vi "Teleop.vi"(10 "Match Info":T2={"Autonomous Elapsed Seconds"=0.0, "TeleOp Elapsed Seconds"=0.0, "Disabled Elapsed Seconds"=0.0, "Visited Autonomous"=FALSE, "Visited TeleOp"=FALSE, "Visited Disabled"=FALSE, "Autonomous Settings"={"Autonomous Style"=enum."Independent", "VI Refnum"=refnum}}, 11 "Call Context":T3) -> ()   [LabVIEW 2016]
doc: "This VI is called for each TeleOp packet received from the DS where the robot is not disabled. It is often used to read from the joysticks and update I/O or to update setpoints for timed control loops. It should complete and return within 20 milliseconds or it may miss DS packets."
uses:
  <vilib>/Rock Robotics/WPI/DriverStation/WPI_DriverStationDerivedRobotMode.ctl
  <vilib>/Rock Robotics/WPI/DriverStation/WPI_DriverStationMatch Info.ctl
  Typedefs/typedef_cluster_Teleop Local Data.ctl
  Typedefs/typedef_enum_Teleop State.ctl
  Typedefs/typedef_enum_Joystick Buttons.ctl
  Robot Global Data.vi
  <vilib>/Rock Robotics/WPI/Utilities/WPI_GetSetVariantRefNum.vi
  <vilib>/Rock Robotics/Network Tables/NT Read Boolean.vi
  <vilib>/Rock Robotics/Network Tables/NT Write Boolean.vi
  <vilib>/Rock Robotics/Network Tables/NT Read Number.vi
  <vilib>/Rock Robotics/WPI/Ultrasonic/WPI_SonarSRF04DigitalRefNum Registry Get.vi
  <vilib>/Rock Robotics/WPI/Ultrasonic/WPI_SonarSRF04DigitalGetRange.vi
panel:
  out "error out":errorcluster
  out "Teleop Local Data out":T1 {"Drive Twist" format="%.2f"; "Drive Forward" format="%.2f"; "Flywheel" format="%.2f"; "Outlet Flap" format="%_4p"; "Inlet Flap" format="%_4p"; "Camera Angle" format="%_4p"; "Collect Motor" format="%_4p"; "Climb Motor" format="%.3f"; "Accel_Y" format="%.3f"; "Accel_X" format="%.3f"; "Obj_deg_Up" format="%.4f"; "Obj_deg_Rt" format="%.1f"; "dT" format="%.4f"}
  out "Sample Slider 0":dbl(slide) scale=0.0..5.0
  out "Sample Boolean 1":bool
  out "Sample Boolean 0":bool
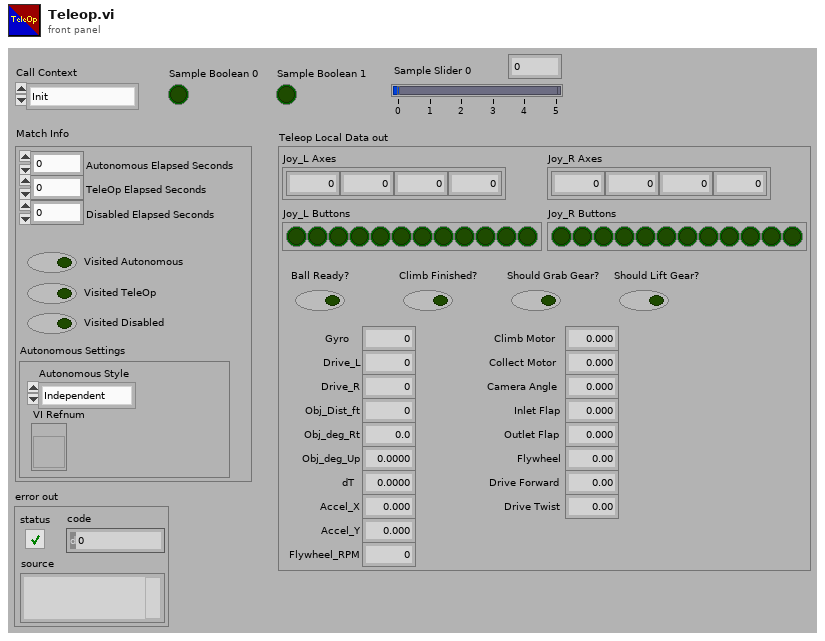
[diagram p1: front panel]
types:
  T1 = typedef "typedef_cluster_Teleop Local Data.ctl" = cluster{"Joy_L Axes":dbl[], "Joy_L Buttons":bool[], "Joy_R Axes":dbl[], "Joy_R Buttons":bool[], "Gyro":dbl, "Drive_L":i32, "Drive_R":i32, "Obj_Dist_ft":dbl, "Obj_deg_Rt":dbl, "Obj_deg_Up":dbl, "dT":dbl, "Accel_X":dbl, "Accel_Y":dbl, "Flywheel_RPM":dbl, "Ball Ready?":bool, "Climb Finished?":bool, "Should Grab Gear?":bool, "Should Lift Gear?":bool, "Climb Motor":dbl, "Collect Motor":dbl, "Camera Angle":dbl, "Inlet Flap":dbl, "Outlet Flap":dbl, "Flywheel":dbl, "Drive Forward":dbl, "Drive Twist":dbl}
  T2 = typedef "WPI_DriverStationMatch Info.ctl" = cluster{"Autonomous Elapsed Seconds":dbl, "TeleOp Elapsed Seconds":dbl, "Disabled Elapsed Seconds":dbl, "Visited Autonomous":bool, "Visited TeleOp":bool, "Visited Disabled":bool, "Autonomous Settings":cluster{"Autonomous Style":enum16{"Iterative", "Independent"}, "VI Refnum":refnum<vi>}}
  T3 = typedef "WPI_DriverStationDerivedRobotMode.ctl" = enum16{"Init", "Execute", "Stop"}
  T4 = typedef "typedef_enum_Teleop State.ctl" = enum16{"StartTeleop", "In Joy_L", "In Joy_R", "In Accel", "In Gyro", "In Drive_L", "In Drive_R", "In Fly_RPMs", "In Switch_Ball", "In Switch_Climbed", "In Get Vision Result", "Calc dT", "Calc Grabber", "Calc Lifter", "Calc Climb", "Calc Collect", "Calc Cam_Angle", "Calc Inlet_Flap", "Calc Outlet_Flap", "Calc Flywheel", "Calc Drive_Forward", "Calc Drive_Twist", "Out Drive_Forward", "Out Drive_Twist", "Out Flywheel", "Out Grabber", "Out Lifter", "Out Climb", "Out Collect", "Out Cam_Angle", "Out Inlet_Flap", "Out Outlet_Flap", "End Teleop"}
  T5 = typedef "typedef_enum_Joystick Buttons.ctl" = enum16{"Trigger", "Thumb", "Top3", "Top4", "Top5", "Top6", "Low7", "Low8", "Low9", "Low10", "Low11", "Low12", "Hat0", "Hat1", "Hat2", "Hat3", "Hat4", "Hat5", "Hat6", "Hat7", "Hat8"}
  T6 = typedef "WPI_JoystickDevRef.ctl" = cluster{"Device":T7}
  T7 = typedef "WPI_JoystickDeviceEnum.ctl" = enum16{"USB 0", "USB 1", "USB 2", "USB 3", "USB 4", "USB 5"}
  T8 = typedef "WPI_AccelerometerDevRef.ctl" = cluster{"DevStatus":errorcluster, "Scaling":T9, "Analog Channels":T10, "I2C Bus":T12, "SPI Bus":T13, "Accel Range":T14, "ADXL Axes":T15, "Handle":i32, "Device Address":u8, "Accel Type":enum16{"Analog", "ADXL345 I2C", "ADXL345 SPI", "Internal", "ADXL362 SPI"}}
  T9 = typedef "WPI_AccelerometerScaling.ctl" = cluster{"Gain (VoltsPerG)":dbl, "Center Voltage":dbl}
  T10 = typedef "WPI_AccelerometerAnalogChannels.ctl" = cluster{"X-Axis":T11, "Y-Axis":T11, "Z-Axis":T11}
  T11 = typedef "FPGA_AIChannel.ctl" = enum8{"AI 0", "AI 1", "AI 2", "AI 3", "AI MXP 0", "AI MXP 1", "AI MXP 2", "AI MXP 3", "Invalid"}
  T12 = typedef "i2c_bus.ctl" = enum16{"I2C On-Board", "I2C MXP", "Invalid"}
  T13 = typedef "spi_bus.ctl" = enum16{"SPI On-Board, CS0", "SPI On-Board, CS1", "SPI On-Board, CS2", "SPI On-Board, CS3", "SPI MXP", "Invalid"}
  T14 = typedef "ADXL345 Range.ctl" = u8
  T15 = typedef "WPI_AccelerometerADXL345 Axes.ctl" = cluster{"X-Axis":bool, "Y-Axis":bool, "Z-Axis":bool}
  T16 = cluster{"X-Axis":dbl, "Y-Axis":dbl, "Z-Axis":dbl}
  T17 = typedef "WPI_GyroDevRef.ctl" = cluster{"DevStatus":errorcluster, "Analog Channel":T11, "Offset":dbl, "Gain (VoltsPerDegree/Second)":dbl, "Gyro Type":enum16{"Analog", "XRS450"}, "Handle":i32, "SPI Bus":T13, "Device Found":bool, "Sample Rate":dbl, "Calibrate On Open":bool}
  T18 = typedef "WPI_MotorControlDeviceRef.ctl" = cluster{"DeviceStatus":errorcluster, "Type":T19, "PWM":cluster{"PWM Channel":T20, "DeadBand":T21}, "CAN":cluster{"Device Number":u8, "SetOutput VI Ref":variant, "GetOutput VI Ref":variant, "Enable VI Ref":variant, "Disable VI Ref":variant, "Data":variant}, "Invert":bool}
  T19 = typedef "WPI_MotorControlType.ctl" = enum16{"PWM", "CAN"}
  T20 = typedef "FPGA_DIOPWMChannel.ctl" = enum8{"PWM 0", "PWM 1", "PWM 2", "PWM 3", "PWM 4", "PWM 5", "PWM 6", "PWM 7", "PWM 8", "PWM 9", "PWM MXP 0", "PWM MXP 1", "PWM MXP 2", "PWM MXP 3", "PWM MXP 4", "PWM MXP 5", "PWM MXP 6", "PWM MXP 7", "PWM MXP 8", "PWM MXP 9", "Invalid"}
  T21 = typedef "WPI_PWMDeadband.ctl" = cluster{"Name":string, "maxPositivePwm":i32, "minPositivePwm":i32, "centerPwm":i32, "maxNegativePwm":i32, "minNegativePwm":i32, "angularRange":u16}
  T22 = typedef "WPI_CANTalonSRX_GlobalStatus.ctl" = cluster{"Applied Throttle":dbl, "Module Enabled":bool, "CAN Error":errorcluster, "Closed Loop Error":dbl, "Forward Limit Switch Closed":bool, "Reverse Limit Switch Closed":bool, "Sensor Position":dbl, "Sensor Velocity":dbl, "Current":dbl, "Sticky Fault - Over Temp":bool, "Sticky Fault - Under Voltage":bool, "Sticky Fault - Forward Limit":bool, "Sticky Fault - Reverse Limit":bool, "Sticky Fault - Forward Soft Limit":bool, "Sticky Fault - Reverse Soft Limit":bool, "Brake is Enabled":bool, "Encoder Position":dbl, "Encoder Velocity":dbl, "Encoder Index Count":dbl, "Encoder A Pin State":bool, "Encoder B Pin State":bool, "Encoder Index Pin State":bool, "Analog In":dbl, "Analog In Velocity":dbl, "Temperature (C)":dbl, "Battery Voltage":dbl, "Control 5 Is Supported":bool, "Current Profile Slot Select":dbl, "Pos Div 8":bool, "Vel Div 4":bool, "Pulse Width Position":i32, "Pulse Width Velocity":i32, "Pulse Width Rise To Rise (us)":i32, "Pulse Width Rise To Fall (us)":i32, "Mot Prof Active Is Under Run":bool, "Mot Prof Active Has Under Run":bool, "Mot Prof Active Is Last":bool, "Mot Prof Active Velocity Only":bool, "Mot Prof Active Is Valid":bool, "Mot Prof Buffer Is Full":bool, "Mot Prof Active Profile Slot Select":i32, "Mot Prof NextID":i32, "Mot Prof Count":i32, "Mot Prof Active Velocity":dbl, "Mot Prof Active Position":dbl, "Mot Prof Output Enable":i32}
  T23 = typedef "WPI_UltrasonicDeviceRef.ctl" = cluster{"DevStatus":errorcluster, "Ping Channel":T24, "Echo Channel":T24, "CntIndex":T25}
  T24 = typedef "FPGA_DIOChannel.ctl" = enum8{"DIO 0", "DIO 1", "DIO 2", "DIO 3", "DIO 4", "DIO 5", "DIO 6", "DIO 7", "DIO 8", "DIO 9", "DIO MXP 0", "DIO MXP 1", "DIO MXP 2", "DIO MXP 3", "DIO MXP 4", "DIO MXP 5", "DIO MXP 6", "DIO MXP 7", "DIO MXP 8", "DIO MXP 9", "DIO MXP 10", "DIO MXP 11", "DIO MXP 12", "DIO MXP 13", "DIO MXP 14", "DIO MXP 15", "SPI Port CS1", "SPI Port CS2", "SPI Port CS3", "SPI Port MISO", "SPI Port MOSI", "Invalid"}
  T25 = typedef "FPGA_CounterCtrSystemIndex.ctl" = enum8{"Ctr 0", "Ctr 1", "Ctr 2", "Ctr 3", "Ctr 4", "Ctr 5", "Ctr 6", "Ctr 7", "Invalid"}
  T26 = typedef "WPI_DigitalInputDevRef.ctl" = cluster{"DevStatus":errorcluster, "DIO Channel":T24}
  T27 = typedef "typedef_cluster_Object Params.ctl" = cluster{"Dist_ft":dbl, "Deg_Rt":dbl, "Deg_Up":dbl, "Cam_FPS":dbl}
  T28 = typedef "WPI_ServoDeviceRef.ctl" = cluster{"DeviceStatus":errorcluster, "PWM Channel":T20, "DeadBand":T21}
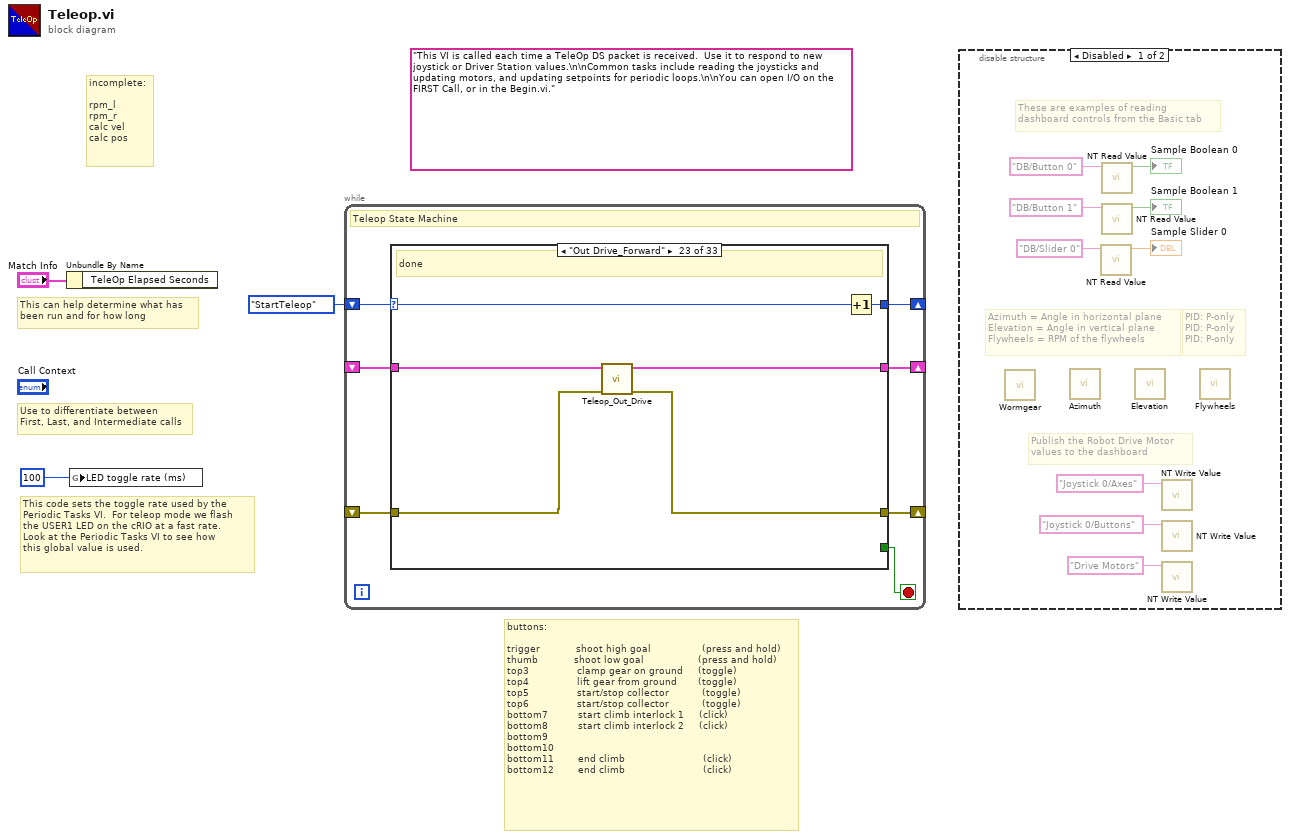
[diagram p0: block diagram]
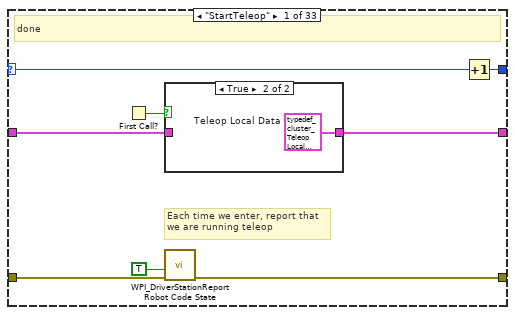
[diagram p3: hidden frame]
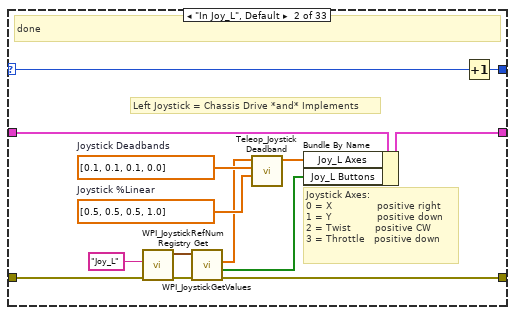
[diagram p5: hidden frame]
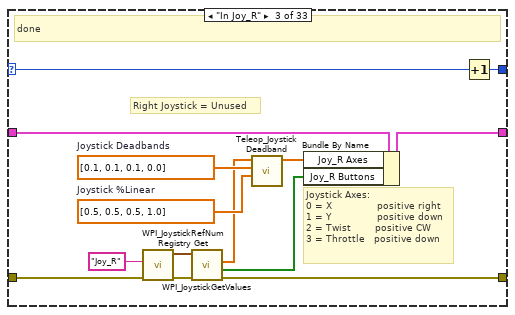
[diagram p6: hidden frame]
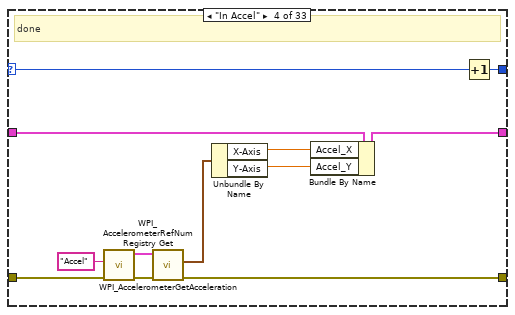
[diagram p7: hidden frame]
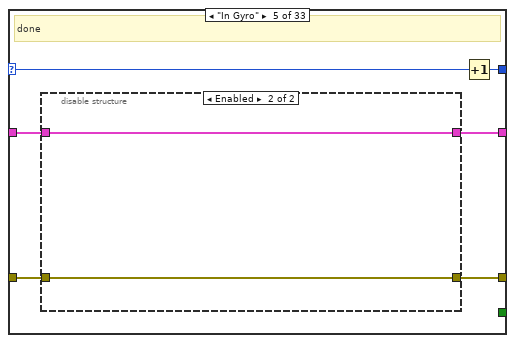
[diagram p8: hidden frame]
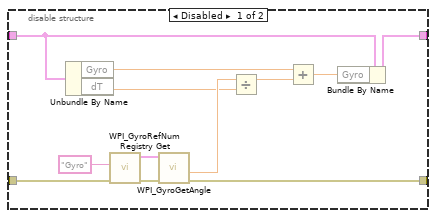
[diagram p9: hidden frame]
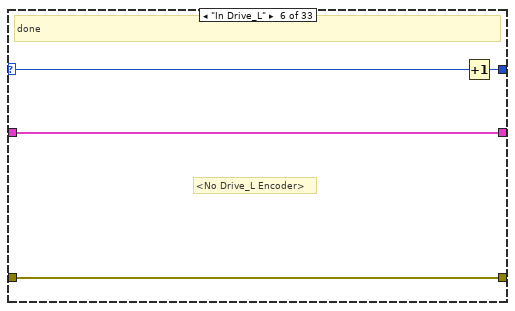
[diagram p10: hidden frame]
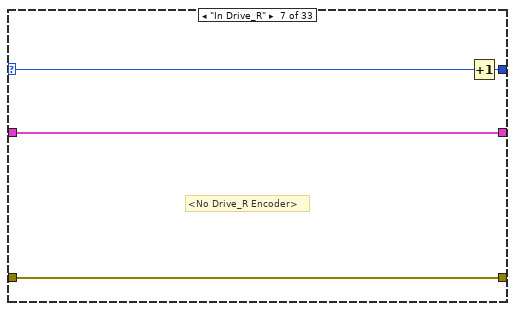
[diagram p11: hidden frame]
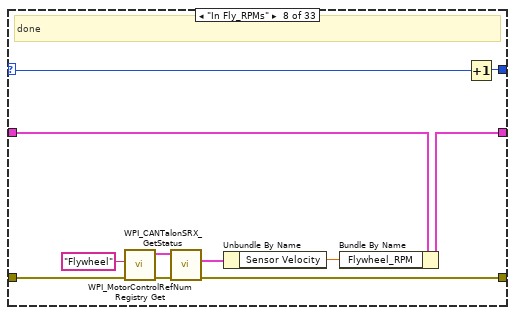
[diagram p12: hidden frame]
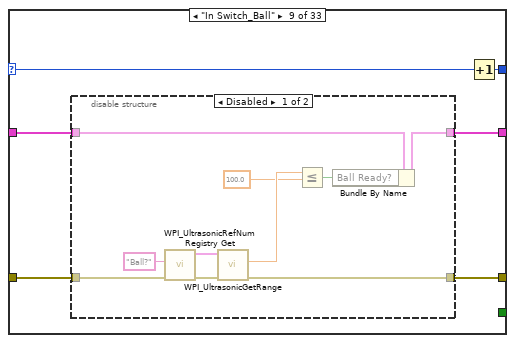
[diagram p13: hidden frame]
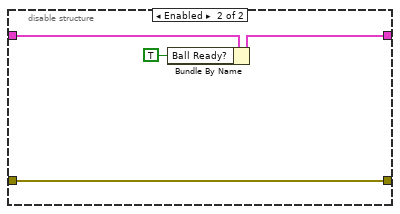
[diagram p14: hidden frame]
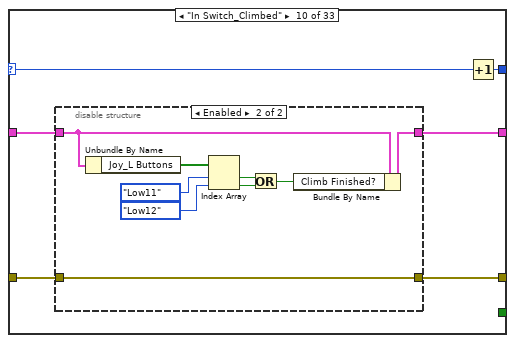
[diagram p15: hidden frame]
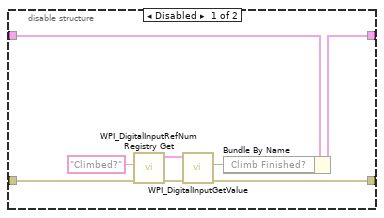
[diagram p16: hidden frame]
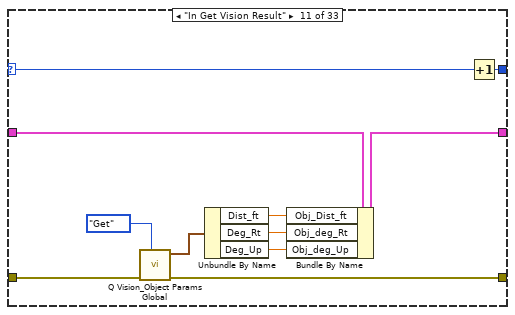
[diagram p17: hidden frame]
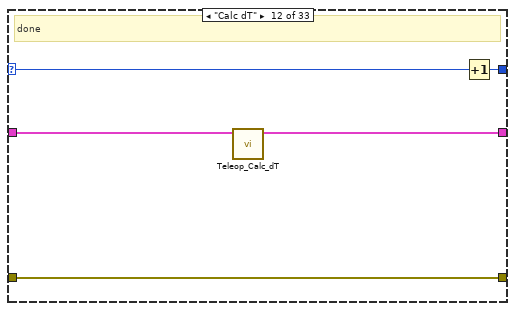
[diagram p18: hidden frame]
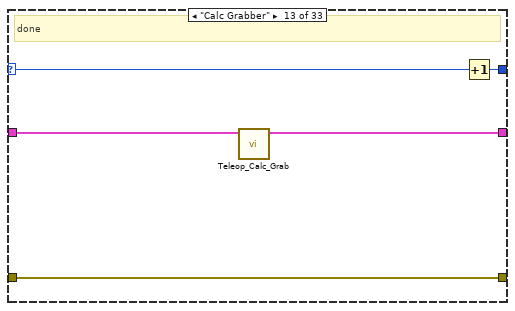
[diagram p19: hidden frame]
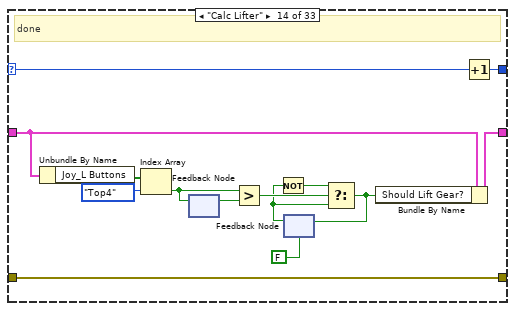
[diagram p20: hidden frame]
diagram:
  (unwired) "This VI is called each time a TeleOp DS packet is received.  Use it to respond to new joystick or Driver Station values.\n\nCommon tasks include reading the joysticks and updating motors, and updating setpoints for periodic loops.\n\nYou can open I/O on the FIRST Call, or in the Begin.vi."
  # "buttons:\n\ntrigger            shoot high goal                \t(press and hold)\nthumb\t\t          shoot low goal \t               \t(press and hold)\ntop3\t\t              clamp gear on ground \t   (toggle)\ntop4\t               lift gear from ground      \t(toggle)\ntop5\t\t              start/stop collector           (toggle)\ntop6\t\t              start/stop collector           (toggle)\nbottom7\t\t        start climb interlock 1    \t(click)\t\nbottom8\t         start climb interlock 2\t    (click)\nbottom9\t\t\nbottom10\t\nbottom11\t       end climb                        \t\t(click)\nbottom12\t       end climb\t\t                        (click)"
  # "incomplete:\n\nrpm_l\nrpm_r\ncalc vel\ncalc pos"
  # "This code sets the toggle rate used by the\nPeriodic Tasks VI.  For teleop mode we flash\nthe USER1 LED on the cRIO at a fast rate. \nLook at the Periodic Tasks VI to see how\nthis global value is used."
  # "Use to differentiate between\nFirst, Last, and Intermediate calls"
  # "This can help determine what has\nbeen run and for how long"
  n1 = Unbundle By Name("Match Info") -> ()  [unwired: 1 out]
  n2 = global write "Robot Global Data.vi" "LED toggle rate (ms)"(u32 100 ("LED ms toggle rate")) -> ()
  n3 = while {
    shift-right: [w10] -> _
    shift-left: typedef_enum_Teleop_State."StartTeleop" ("Teleop State") -> [w4]
    shift-right: [w6] -> _
    shift-left: _ -> [w7]
    shift-right: [w8] -> _
    shift-left: _ -> [w9]
    stop <- w5 stop-if-true
    # "Teleop State Machine"
    n4 = case shown="\"Out Drive_Forward\"" w4 {
      selector: w4 -> [w18 w33 w47 w60 w66 w84 w86 w91 w104 w124 w152 w158 w163 w177 w182 w187 w191 w196 w207 w212 w217 w222 w228 w232 w238 w244 w250 w256 w261 w265 w268 w283 w289]
      tunnel: [w17 w32 w46 w59 w65 w83 w85 w92 w105 w125 w153 w157 w162 w176 w181 w186 w190 w195 w206 w211 w216 w221 w227 w231 w237 w243 w249 w255 w262 w266 w267 w284 w288] -> w10
      tunnel: w9 -> [w12 w28 w42 w52 w63 w82 w87 w90 w101 w120 w151 w156 w159 w173 w180 w185 w189 w194 w205 w210 w215 w220 w226 w229 w234 w240 w246 w252 w258 w263 w273 w279 w285]
      tunnel: [w11 w27 w41 w53 w62 w82 w87 w89 w100 w121 w150 w156 w159 w173 w180 w185 w189 w194 w205 w210 w215 w220 w225 w229 w233 w239 w245 w251 w257 w263 w272 w278 w285] -> w8
      tunnel: w7 -> [w14 w24 w38 w58 w61 w81 w88 w95 w103 w123 w148 w155 w160 w174 w179 w184 w188 w192 w197 w209 w214 w218 w224 w230 w236 w242 w248 w254 w260 w264 w269 w277 w287]
      tunnel: [w16 w26 w40 w51 w64 w81 w88 w93 w102 w122 w147 w154 w161 w175 w178 w183 w188 w193 w202 w208 w213 w219 w223 w230 w235 w241 w247 w253 w259 w264 w269 w277 w287] -> w6
      tunnel: [_ _ _ _ _ _ _ _ _ _ _ _ _ _ _ _ _ _ _ _ _ _ _ _ _ _ _ _ _ _ _ _ w286] -> w5
      frame "StartTeleop" {
        # "Each time we enter, report that\nwe are running teleop"
        # "done"
        n5 = First Call?() -> (First Call?: T/F=w15:bool)
        n6 = case shown="True" w15 {
          tunnel: [w19 w20] -> w16
          tunnel: w14 -> [w19 _]
          frame False {
          }
          frame True {
            w20 = T1 {"Joy_L Axes"=[], "Joy_L Buttons"=[], "Joy_R Axes"=[], "Joy_R Buttons"=[], "Gyro"=0.0, "Drive_L"=0, "Drive_R"=0, "Obj_Dist_ft"=0.0, "Obj_deg_Rt"=0.0, "Obj_deg_Up"=0.0, "dT"=0.0, "Accel_X"=0.0, "Accel_Y"=0.0, "Flywheel_RPM"=0.0, "Ball Ready?"=FALSE, "Climb Finished?"=FALSE, "Should Grab Gear?"=FALSE, "Should Lift Gear?"=FALSE, "Climb Motor"=0.0, "Collect Motor"=0.0, "Camera Angle"=0.0, "Inlet Flap"=0.0, "Outlet Flap"=0.0, "Flywheel"=0.0, "Drive Forward"=0.0, "Drive Twist"=0.0}  # Teleop Local Data
          }
        }
        n7 = call <vilib>:"WPI_DriverStationReport Robot Code State.vi"("error in (no error)"=w12, "TeleOp"=TRUE ("Autonomous")) -> ("error out"=w11:errorcluster)  [unwired: 9 in]
        n8 = Increment(x=w18) -> (x+1=w17:T4)
      }
      frame "In Joy_L", Default {
        w34 = dbl[] [0.5, 0.5, 0.5, 1.0]  # Joystick %Linear
        w23 = dbl[] [0.1, 0.1, 0.1, 0.0]  # Joystick Deadbands
        # "Left Joystick = Chassis Drive *and* Implements"
        # "Joystick Axes:\n0 = X               positive right\n1 = Y               positive down\n2 = Twist        positive CW\n3 = Throttle   positive down"
        # "done"
        n9 = call <vilib>:"WPI_JoystickRefNum Registry Get.vi"("error in (no error)"=w28, "refnum name"="Joy_L") -> ("error out"=w31:errorcluster, "JoystickDevRef"=w30:T6)  [unwired: 8 out]
        n10 = call <vilib>:"WPI_JoystickGetValues.vi"("error in (no error)"=w31, "JoystickDevRef"=w30) -> ("error out"=w27:errorcluster, "Buttons"=w25:bool[], "Axes"=w22:dbl[])  [unwired: 5 in, 2 out]
        n11 = call "Teleop_Joystick Deadband.vi"("Joystick %Linear"=w34, "Joystick Deadbands"=w23, "Joystick Axes in"=w22) -> ("Joystick Axes out"=w21:dbl[])  [unwired: 8 in]
        n12 = Bundle By Name(cluster=w24, "Joy_L Axes"=w21, "Joy_L Buttons"=w25) -> (w26:T1)
        n13 = Increment(x=w33) -> (x+1=w32:T4)
      }
      frame "In Joy_R" {
        w48 = dbl[] [0.5, 0.5, 0.5, 1.0]  # Joystick %Linear
        w37 = dbl[] [0.1, 0.1, 0.1, 0.0]  # Joystick Deadbands
        # "Right Joystick = Unused"
        # "Joystick Axes:\n0 = X               positive right\n1 = Y               positive down\n2 = Twist        positive CW\n3 = Throttle   positive down"
        # "done"
        n14 = call <vilib>:"WPI_JoystickRefNum Registry Get.vi"("error in (no error)"=w42, "refnum name"="Joy_R") -> ("error out"=w45:errorcluster, "JoystickDevRef"=w44:T6)  [unwired: 8 out]
        n15 = call <vilib>:"WPI_JoystickGetValues.vi"("error in (no error)"=w45, "JoystickDevRef"=w44) -> ("error out"=w41:errorcluster, "Buttons"=w39:bool[], "Axes"=w36:dbl[])  [unwired: 5 in, 2 out]
        n16 = call "Teleop_Joystick Deadband.vi"("Joystick %Linear"=w48, "Joystick Deadbands"=w37, "Joystick Axes in"=w36) -> ("Joystick Axes out"=w35:dbl[])  [unwired: 8 in]
        n17 = Bundle By Name(cluster=w38, "Joy_R Axes"=w35, "Joy_R Buttons"=w39) -> (w40:T1)
        n18 = Increment(x=w47) -> (x+1=w46:T4)
      }
      frame "In Accel" {
        # "done"
        n19 = call <vilib>:"WPI_AccelerometerRefNum Registry Get.vi"("error in (no error)"=w52, "refnum name"="Accel") -> ("error out"=w56:errorcluster, "AccelerometerDevRef"=w55:T8)  [unwired: 8 in]
        n20 = call <vilib>:"WPI_AccelerometerGetAcceleration.vi"("error in"=w56, "AccelerometerDevRef"=w55) -> ("error out"=w53:errorcluster, "Accelerations"=w54:T16)  [unwired: 7 in, 1 out]
        n21 = Unbundle By Name(w54) -> ("X-Axis"=w50:dbl, "Y-Axis"=w49:dbl)
        n22 = Bundle By Name(cluster=w58, "Accel_X"=w50, "Accel_Y"=w49) -> (w51:T1)
        n23 = Increment(x=w60) -> (x+1=w59:T4)
      }
      frame "In Gyro" {
        # "done"
        n24 = disable-structure shown="Enabled" {
          disable-tunnel: [w78 w80] -> w64
          disable-tunnel: w63 -> [w74 w79]
          disable-tunnel: [w73 w79] -> w62
          disable-tunnel: w61 -> [w72 w80]
          frame Disabled {
            n25 = Unbundle By Name(w72) -> ("Gyro"=w70:dbl, "dT"=w67:dbl)
            n26 = call <vilib>:"WPI_GyroRefNum Registry Get.vi"("error in (no error)"=w74, "refnum name"="Gyro") -> ("error out"=w75:errorcluster, "GyroDevRef"=w76:T17)  [unwired: 8 in]
            n27 = call <vilib>:"WPI_GyroGetAngle.vi"("error in"=w75, "GyroDevRef"=w76) -> ("error out"=w73:errorcluster, "Angular Rate"=w69:dbl)  [unwired: 5 in, 3 out]
            n28 = Divide(x=w69, y=w67) -> (x/y=w68:dbl)
            n29 = Add(x=w70, y=w68) -> (x+y=w71:dbl)
            n30 = Bundle By Name(cluster=w72, "Gyro"=w71) -> (w78:T1)
          }
          frame Enabled {
          }
        }
        n31 = Increment(x=w66) -> (x+1=w65:T4)
      }
      frame "In Drive_L" {
        # "<No Drive_L Encoder>"
        # "done"
        n32 = Increment(x=w84) -> (x+1=w83:T4)
      }
      frame "In Drive_R" {
        # "<No Drive_R Encoder>"
        n33 = Increment(x=w86) -> (x+1=w85:T4)
      }
      frame "In Fly_RPMs" {
        # "done"
        n34 = call <vilib>:"WPI_MotorControlRefNum Registry Get.vi"("error in (no error)"=w90, "refnum name"="Flywheel") -> ("error out"=w99:errorcluster, "MotorControlDevRef"=w98:T18)  [unwired: 8 in]
        n35 = call <vilib>:"WPI_CANTalonSRX_GetStatus.vi"("error in (no error)"=w99, "CAN Talon SRX Ref"=w98) -> ("error out"=w89:errorcluster, "Talon SRX Status"=w96:T22)  [unwired: 7 in, 1 out]
        n36 = Unbundle By Name(w96) -> ("Sensor Velocity"=w94:dbl)
        n37 = Bundle By Name(cluster=w95, "Flywheel_RPM"=w94) -> (w93:T1)
        n38 = Increment(x=w91) -> (x+1=w92:T4)
      }
      frame "In Switch_Ball" {
        n39 = disable-structure shown="Disabled" {
          disable-tunnel: w103 -> [w113 w118]
          disable-tunnel: [w112 w117] -> w102
          disable-tunnel: w101 -> [w107 w119]
          disable-tunnel: [w106 w119] -> w100
          frame Disabled {
            n40 = call-poly <vilib>:"WPI_UltrasonicRefNum Registry Get.vi"("error in (no error)"=w107, "refnum name"="Ball?") -> ("error out"=w114:errorcluster, "SonarSRF04DevRef"=w115:T23)  [unwired: 8 in]
            n41 = call-poly <vilib>:"WPI_UltrasonicGetRange.vi"("error in (no error)"=w114, "SonarSRF04DevRef"=w115) -> ("error out"=w106:errorcluster, "Distance"=w110:dbl)  [unwired: 7 in, 1 out]
            n42 = Less Or Equal?(x=w110, y=100.0) -> (x <= y?=w109:bool)
            n43 = Bundle By Name(cluster=w113, "Ball Ready?"=w109) -> (w112:T1)
          }
          frame Enabled {
            n44 = Bundle By Name(cluster=w118, "Ball Ready?"=TRUE) -> (w117:T1)
          }
        }
        n45 = Increment(x=w104) -> (x+1=w105:T4)
      }
      frame "In Switch_Climbed" {
        n46 = disable-structure shown="Enabled" {
          disable-tunnel: w123 -> [w129 w140]
          disable-tunnel: [w128 w141] -> w122
          disable-tunnel: [w127 w142] -> w121
          disable-tunnel: w120 -> [w126 w142]
          frame Disabled {
            n47 = call <vilib>:"WPI_DigitalInputRefNum Registry Get.vi"("error in (no error)"=w126, "refnum name"="Climbed?") -> ("error out"=w132:errorcluster, "DigitalInputDevRef"=w130:T26)  [unwired: 8 in]
            n48 = call <vilib>:"WPI_DigitalInputGetValue.vi"("error in (no error)"=w132, "DigitalInputDevRef"=w130) -> ("error out"=w127:errorcluster, "Value"=w131:bool)  [unwired: 7 in, 1 out]
            n49 = Bundle By Name(cluster=w129, "Climb Finished?"=w131) -> (w128:T1)
          }
          frame Enabled {
            n50 = Unbundle By Name(w140) -> ("Joy_L Buttons"=w137:bool[])
            n51 = Index Array(array=w137, index #1=typedef_enum_Joystick_Buttons."Low11" ("Joystick Buttons"), index #2=typedef_enum_Joystick_Buttons."Low12" ("Joystick Buttons")) -> (element #1=w136:bool, element #2=w135:bool)
            n52 = Or(x=w136, y=w135) -> (x .or. y?=w134:bool)
            n53 = Bundle By Name(cluster=w140, "Climb Finished?"=w134) -> (w141:T1)
          }
        }
        n54 = Increment(x=w124) -> (x+1=w125:T4)
      }
      frame "In Get Vision Result" {
        n55 = call "Q Vision_Object Params Global.vi"("Action"=enum16{"Get", "Set"}."Get", "error in (no error)"=w151) -> ("error out"=w150:errorcluster, "Object Params out"=w146:T27)  [unwired: 8 in]
        n56 = Unbundle By Name(w146) -> ("Dist_ft"=w145:dbl, "Deg_Rt"=w144:dbl, "Deg_Up"=w143:dbl)
        n57 = Bundle By Name(cluster=w148, "Obj_Dist_ft"=w145, "Obj_deg_Rt"=w144, "Obj_deg_Up"=w143) -> (w147:T1)
        n58 = Increment(x=w152) -> (x+1=w153:T4)
      }
      frame "Calc dT" {
        # "done"
        n59 = call "Teleop_Calc_dT.vi"("Teleop Local Data in"=w155) -> ("Teleop Local Data out"=w154:T1)  [unwired: 10 in]
        n60 = Increment(x=w158) -> (x+1=w157:T4)
      }
      frame "Calc Grabber" {
        # "done"
        n61 = call "Teleop_Calc_Grab.vi"("Teleop Local Data in"=w160) -> ("Teleop Local Data out"=w161:T1)  [unwired: 10 in]
        n62 = Increment(x=w163) -> (x+1=w162:T4)
      }
      frame "Calc Lifter" {
        # "done"
        n63 = Unbundle By Name(w174) -> ("Joy_L Buttons"=w172:bool[])
        n64 = Index Array(array=w172, index=typedef_enum_Joystick_Buttons."Top4" ("Joystick Buttons")) -> (element=w164:bool)
        n65 = feedback #1() -> (w170:bool)  [unwired: 1 in]
        n66 = feedback-in #1(w164) -> ()
        n67 = Greater?(x=w164, y=w170) -> (0:w169:bool)
        n68 = feedback #2(FALSE) -> (w167:bool)
        n69 = Not(x=w167) -> (.not. x?=w166:bool)
        n70 = Select(t=w166, s=w169, f=w167) -> (s? t:f=w165:bool)
        n71 = feedback-in #2(w165) -> ()
        n72 = Bundle By Name(cluster=w174, "Should Lift Gear?"=w165) -> (w175:T1)
        n73 = Increment(x=w177) -> (x+1=w176:T4)
      }
      frame "Calc Climb" {
        # "done"
        n74 = call "Teleop_Calc_Climb.vi"("Teleop Local Data in"=w179) -> ("Teleop Local Data out"=w178:T1)  [unwired: 10 in]
        n75 = Increment(x=w182) -> (x+1=w181:T4)
      }
      frame "Calc Collect" {
        # "done"
        n76 = call "Teleop_Calc_Collect.vi"("Teleop Local Data in"=w184) -> ("Teleop Local Data out"=w183:T1)  [unwired: 10 in]
        n77 = Increment(x=w187) -> (x+1=w186:T4)
      }
      frame "Calc Cam_Angle" {
        # "Finished"
        # "done"
        n78 = Increment(x=w191) -> (x+1=w190:T4)
      }
      frame "Calc Inlet_Flap" {
        # "done"
        n79 = call "Teleop_Calc_Inlet.vi"("Teleop Local Data in"=w192) -> ("Teleop Local Data out"=w193:T1)  [unwired: 10 in]
        n80 = Increment(x=w196) -> (x+1=w195:T4)
      }
      frame "Calc Outlet_Flap" {
        # "done"
        n81 = Unbundle By Name(w197) -> ("Joy_L Buttons"=w203:bool[])
        n82 = Index Array(array=w203, index=typedef_enum_Joystick_Buttons."Thumb" ("Joystick Buttons")) -> (element=w201:bool)
        n83 = Select(t=0.5, s=w201, f=0.0) -> (s? t:f=w200:dbl)
        n84 = Bundle By Name(cluster=w197, "Outlet Flap"=w200) -> (w202:T1)
        n85 = Increment(x=w207) -> (x+1=w206:T4)
      }
      frame "Calc Flywheel" {
        # "done"
        n86 = call "Teleop_Calc_Flywheel.vi"("Teleop Local Data in"=w209) -> ("Teleop Local Data out"=w208:T1)  [unwired: 10 in]
        n87 = Increment(x=w212) -> (x+1=w211:T4)
      }
      frame "Calc Drive_Forward" {
        # "done"
        n88 = call "Teleop_Calc_Forward.vi"("Teleop Local Data in"=w214) -> ("Teleop Local Data out"=w213:T1)  [unwired: 10 in]
        n89 = Increment(x=w217) -> (x+1=w216:T4)
      }
      frame "Calc Drive_Twist" {
        # "done"
        n90 = call "Teleop_Calc_Drive_Twist.vi"("Teleop Local Data in"=w218) -> ("Teleop Local Data out"=w219:T1)  [unwired: 10 in]
        n91 = Increment(x=w222) -> (x+1=w221:T4)
      }
      frame "Out Drive_Forward" {
        # "done"
        n92 = call "Teleop_Out_Drive.vi"("error in (no error)"=w226, "Teleop Local Data in"=w224) -> ("error out"=w225:errorcluster, "Teleop Local Data out"=w223:T1)  [unwired: 8 in]
        n93 = Increment(x=w228) -> (x+1=w227:T4)
      }
      frame "Out Drive_Twist" {
        # "done"
        n94 = Increment(x=w232) -> (x+1=w231:T4)
      }
      frame "Out Flywheel" {
        # "done"
        n95 = call "Teleop_Out_Flywheel.vi"("error in (no error)"=w234, "Teleop Local Data in"=w236) -> ("error out"=w233:errorcluster, "Teleop Local Data Out"=w235:T1)  [unwired: 8 in]
        n96 = Increment(x=w238) -> (x+1=w237:T4)
      }
      frame "Out Grabber" {
        # "done"
        n97 = call "Teleop_Out_Grabber.vi"("error in (no error)"=w240, "Teleop Local Data Out"=w242) -> ("error out"=w239:errorcluster, "Teleop Local Data Out 2"=w241:T1)  [unwired: 8 in]
        n98 = Increment(x=w244) -> (x+1=w243:T4)
      }
      frame "Out Lifter" {
        # "done"
        n99 = call "Teleop_Out_Lifter.vi"("error in (no error)"=w246, "Teleop Local Data Out"=w248) -> ("error out"=w245:errorcluster, "Teleop Local Data Out 2"=w247:T1)  [unwired: 8 in]
        n100 = Increment(x=w250) -> (x+1=w249:T4)
      }
      frame "Out Climb" {
        # "done"
        n101 = call "Teleop_Out_Climb.vi"("error in (no error)"=w252, "Teleop Local Data Out"=w254) -> ("error out"=w251:errorcluster, "Teleop Local Data Out 2"=w253:T1)  [unwired: 8 in]
        n102 = Increment(x=w256) -> (x+1=w255:T4)
      }
      frame "Out Collect" {
        n103 = call "Teleop_Out_Collect.vi"("error in (no error)"=w258, "Teleop Local Data Out"=w260) -> ("error out"=w257:errorcluster, "Teleop Local Data Out 2"=w259:T1)  [unwired: 8 in]
        n104 = Increment(x=w261) -> (x+1=w262:T4)
      }
      frame "Out Cam_Angle" {
        n105 = Increment(x=w265) -> (x+1=w266:T4)
      }
      frame "Out Inlet_Flap" {
        n106 = Unbundle By Name(w269) -> ("Inlet Flap"=w270:dbl)
        n107 = call <vilib>:"WPI_ServoRefNum Registry Get.vi"("error in (no error)"=w273, "refnum name"="Inlet_Flap") -> ("error out"=w274:errorcluster, "ServoDeviceRef"=w275:T28)  [unwired: 8 in]
        n108 = call <vilib>:"WPI_ServoSetPosition.vi"("error in (no error)"=w274, "Position"=w270, "ServoDeviceRef"=w275) -> ("error out"=w272:errorcluster)  [unwired: 7 in, 1 out]
        n109 = Increment(x=w268) -> (x+1=w267:T4)
      }
      frame "Out Outlet_Flap" {
        n110 = Unbundle By Name(w277) -> ("Outlet Flap"=w276:dbl)
        n111 = call <vilib>:"WPI_ServoRefNum Registry Get.vi"("error in (no error)"=w279, "refnum name"="Outlet_Flap") -> ("error out"=w281:errorcluster, "ServoDeviceRef"=w282:T28)  [unwired: 8 in]
        n112 = call <vilib>:"WPI_ServoSetPosition.vi"("error in (no error)"=w281, "Position"=w276, "ServoDeviceRef"=w282) -> ("error out"=w278:errorcluster)  [unwired: 7 in, 1 out]
        n113 = Increment(x=w283) -> (x+1=w284:T4)
      }
      frame "End Teleop" {
        w286 = TRUE  # Last Step!
        # "done"
        n114 = Increment(x=w289) -> (x+1=w288:T4)
        "Teleop Local Data out" <- w287
        "error out" <- w285
      }
    }
  }
  n115 = disable-structure shown="Disabled" {
    frame Disabled {
      # "These are examples of reading\ndashboard controls from the Basic tab"
      # "Publish the Robot Drive Motor\nvalues to the dashboard"
      # "PID: P-only\nPID: P-only\nPID: P-only"
      # "Azimuth = Angle in horizontal plane\nElevation = Angle in vertical plane\nFlywheels = RPM of the flywheels"
      n116 = call "Wormgear.vi"() -> ()  [unwired: 10 in, 2 out]
      n117 = call "Azimuth.vi"() -> ()  [unwired: 12 in, 4 out]
      n118 = call-poly <vilib>:"NT Read Value.vi"("Name"="DB/Slider 0" ("refnum name")) -> ("Numeric"=→"Sample Slider 0":dbl)  [unwired: 9 in, 1 out]
      n119 = call-poly <vilib>:"NT Read Value.vi"("Name"="DB/Button 0" ("refnum name")) -> ("Boolean"=→"Sample Boolean 0":bool)  [unwired: 9 in, 1 out]
      n120 = call-poly <vilib>:"NT Read Value.vi"("Name"="DB/Button 1" ("refnum name")) -> ("Boolean"=→"Sample Boolean 1":bool)  [unwired: 9 in, 1 out]
      n121 = call "Elevation.vi"() -> ()  [unwired: 12 in, 4 out]
      n122 = call-poly <vilib>:"NT Write Value.vi"("Name"="Joystick 0/Axes") -> ()  [unwired: 10 in, 1 out]
      n123 = call-poly <vilib>:"NT Write Value.vi"("Name"="Joystick 0/Buttons") -> ()  [unwired: 10 in, 1 out]
      n124 = call-poly <vilib>:"NT Write Value.vi"("Name"="Drive Motors") -> ()  [unwired: 10 in, 1 out]
      n125 = call "Flywheels.vi"() -> ()  [unwired: 12 in, 4 out]
    }
    frame Enabled {
    }
  }
